vi "action.vi"(0 "HB_Simple_Increment":refnum<class "HB_Simple_Decrement.lvclass">, 2 "HGF_Visitable":refnum<class "HGF_Visitable.lvclass">, 5 "error in (no error)":errorcluster) -> (14 "dup HB_Simple_Increment":refnum<class "HB_Simple_Decrement.lvclass">, 16 "dup HGF_Visitable":refnum<class "HGF_Visitable.lvclass">, 19 "error out":errorcluster)   [LabVIEW 2009, in "HB_BaseClass_Examples.lvlib" / "HB_Simple_Decrement.lvclass"]
doc: "This is a dynamic dispatch VI that is called from Visitor.visit(). It will call member VIs of Visitable to perform the requested action which means: calling public methods of Visitable child class.\n\n<B>Hint:</B> This method is abstract and need to be implemented by child classes."
uses:
  HB_Simple_Decrement.lvclass
  lib.lib/HGF_LVC/HGF_BaseClasses/HGF_Visitable/HGF_Visitable.lvclass
  HB_Simple.lvclass
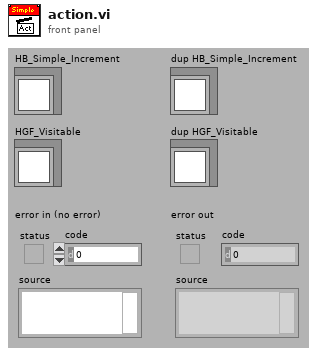
[diagram p1: front panel]
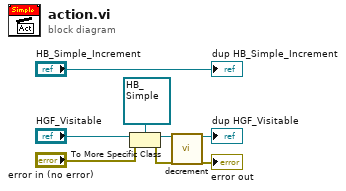
[diagram p0: block diagram]
diagram:
  n1 = To More Specific Class(target class=refnum<class "HB_Simple.lvclass"> refnum ("HB_Simple.lvclass"), reference="HGF_Visitable", error in="error in (no error)") -> (specific class reference=w4:refnum<class "HB_Simple.lvclass">, error out=w2:errorcluster)
  n2 = call "decrement.vi"("HB_Simple in"=w4, "error in (no error)"=w2) -> ("HB_Simple out"=→"dup HGF_Visitable":refnum<class "HB_Simple.lvclass">, "error out"=→"error out":errorcluster)  [unwired: 16 out]
  "dup HB_Simple_Increment" <- "HB_Simple_Increment"
